vi "process tdms folder.vi"() -> ()   [LabVIEW 2021]
uses:
  NHMFL_Core/Libraries/File/File Format Converter/Format Converter Configuration.ctl
  <vilib>/Utility/TDMS File Viewer/NI_TDMS File Viewer.lvlib
  nanocal_process_tdms_file_control.ctl
panel:
  out "current file index":i32
  out "current file":path
  out "# of files":i32
  out "All Files in Dir":path[](array[path])
  out "ALL channel names":string[](array[string])
  out "new Configuration":T1={"New start time"=nan, "New end time"=nan, "Output file format"=enum."ASCII", "Save ASCII column names"=TRUE, "Prepend binary array size"=FALSE, "buffer size (-1: all)"=100000, "Group"="p", "New dt"=nan, "IGORify column names"=TRUE, "eliminate spaces in col name"=TRUE, "Channels"=[]} {"buffer size (-1: all)" format="%.0p"; "New start time" format="%#_10p"}
  in  "pattern":string="m*_*.tdms"
  in  "Configuration":T1={"New start time"=nan, "New end time"=nan, "Output file format"=enum."ASCII", "Save ASCII column names"=TRUE, "Prepend binary array size"=FALSE, "buffer size (-1: all)"=100000, "Group"="p", "New dt"=nan, "IGORify column names"=TRUE, "eliminate spaces in col name"=TRUE, "Channels"=["jsdhgv", "lsjdfh", "ajlsd"]} {"buffer size (-1: all)" format="%.0p"; "New start time" format="%#_10p"}
  in  "Folder Path":path=path "/Users/arkadyshekhter/Library/CloudStorage/Dropbox/shared_Ali/nanocal-March2020 - RuCl3/March_2020"
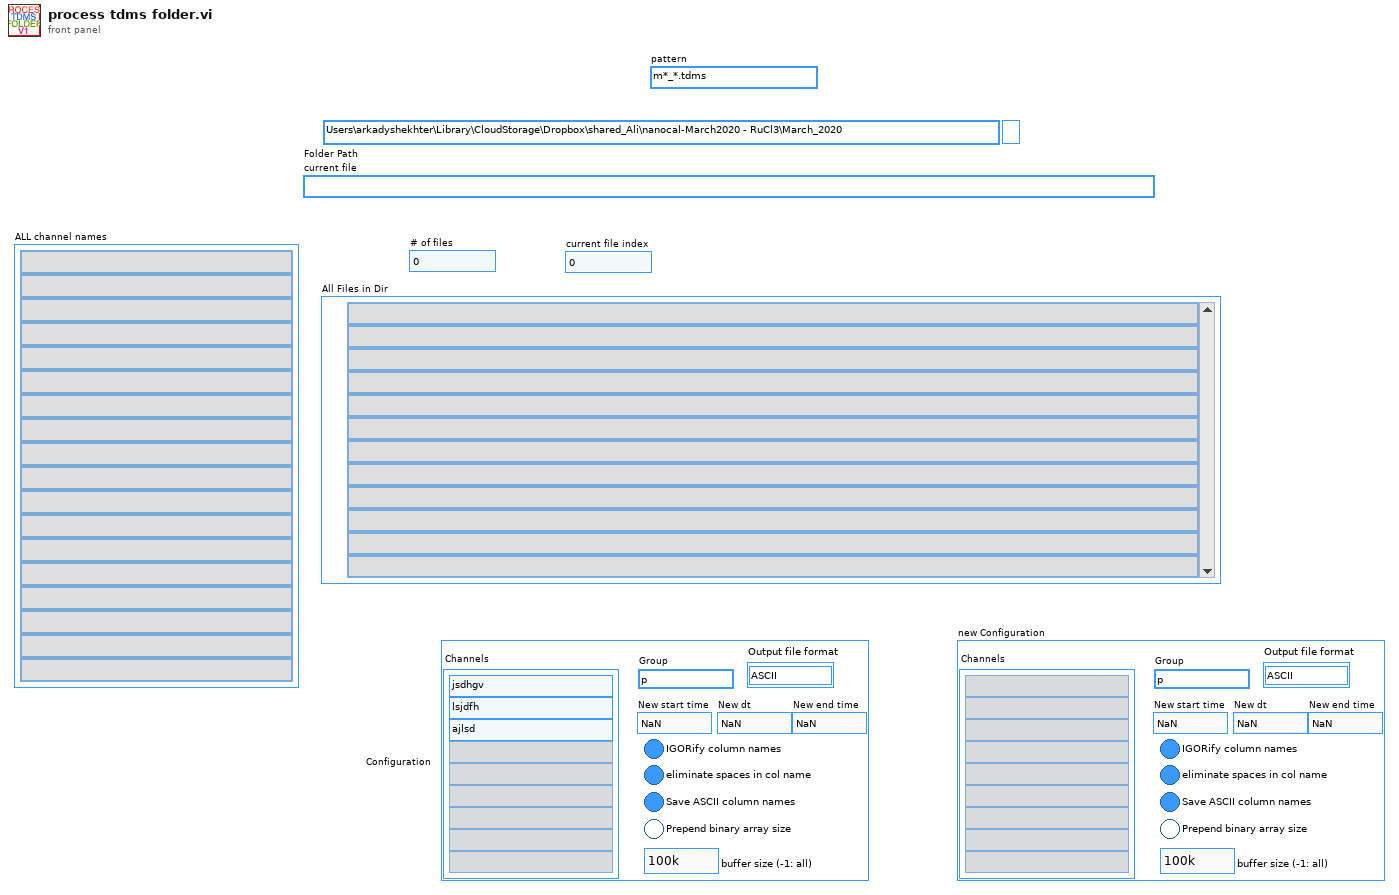
[diagram p1: front panel]
types:
  T1 = typedef "Format Converter Configuration.ctl" = cluster{"New start time":dbl, "New end time":dbl, "Output file format":enum16{"ASCII", "BINARY", "TDMS"}, "Save ASCII column names":bool, "Prepend binary array size":bool, "buffer size (-1: all)":i64, "Group":string, "New dt":dbl, "IGORify column names":bool, "eliminate spaces in col name":bool, "Channels":string[]}
  T2 = typedef "nanocal_process_tdms_file_control.ctl" = enum16{"all fileds", "subset of fields"}
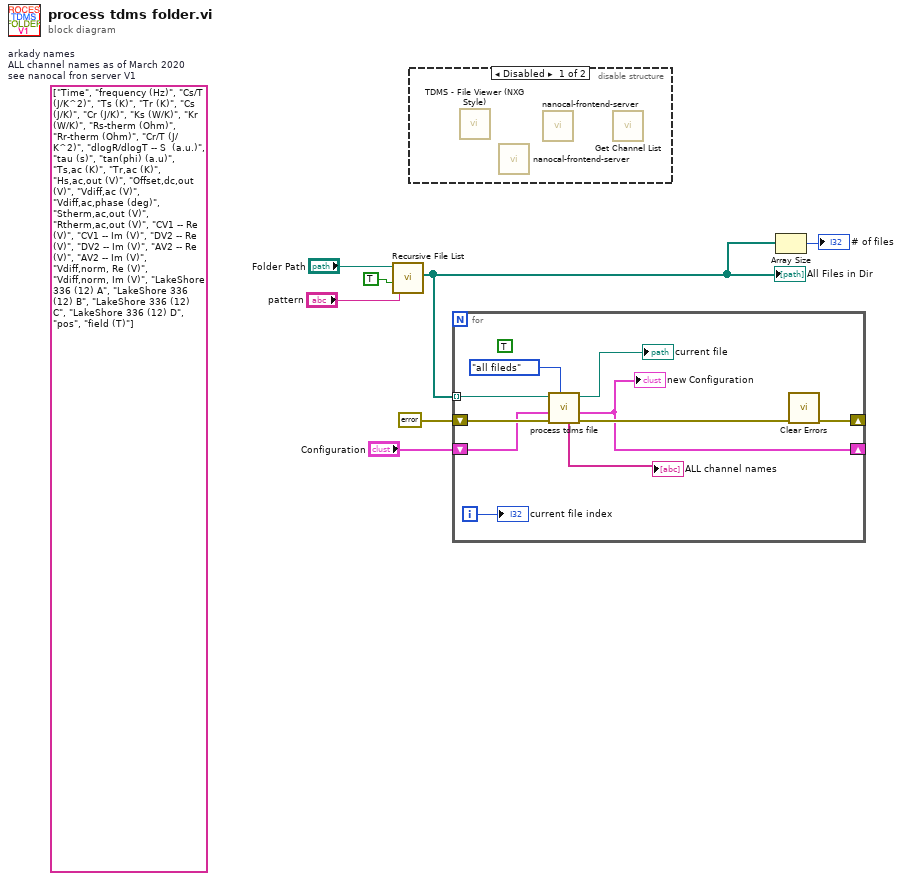
[diagram p0: block diagram]
diagram:
  (unwired) string[] ["Time", "frequency (Hz)", "Cs/T (J/K^2)", "Ts (K)", "Tr (K)", "Cs (J/K)", "Cr (J/K)", "Ks (W/K)", "Kr (W/K)", "Rs-therm (Ohm)", "Rr-therm (Ohm)", "Cr/T (J/K^2)", "dlogR/dlogT -- S  (a.u.)", "tau (s)", "tan(phi) (a.u)", "Ts,ac (K)", "Tr,ac (K)", "Hs,ac,out (V)", "Offset,dc,out (V)", "Vdiff,ac (V)", "Vdiff,ac,phase (deg)", "Stherm,ac,out (V)", "Rtherm,ac,out (V)", "CV1 -- Re (V)", "CV1 -- Im (V)", "DV2 -- Re (V)", "DV2 -- Im (V)", "AV2 -- Re (V)", "AV2 -- Im (V)", "Vdiff,norm, Re (V)", "Vdiff,norm, Im (V)", "LakeShore 336 (12) A", "LakeShore 336 (12) B", "LakeShore 336 (12) C", "LakeShore 336 (12) D", "pos", "field (T)"]  # arkady names ALL channel names as of March 2020 see nanocal fron server V1
  n1 = call <vilib>:"Recursive File List.vi"("pattern"="pattern", "Continue Recursing on Error? (F)"=TRUE, "Folder Path"="Folder Path") -> ("All Files in Dir"=w1:path[])  [unwired: 4 in, 4 out]
  "All Files in Dir" <- w1
  n2 = disable-structure shown="Disabled" {
    frame Disabled {
      n3 = call <vilib>:"TDMS - File Viewer (NXG Style).vi"() -> ()  [unwired: 10 in, 2 out]
      n4 = call "nanocal-frontend-server.vi"() -> ()  [unwired: 12 in]
      n5 = call "nanocal-frontend-server.vi"() -> ()  [unwired: 12 in]
      n6 = call <vilib>:"Get Channel List.vi"() -> ()  [unwired: 5 in, 3 out]
    }
    frame Enabled {
    }
  }
  n7 = for {
    tunnel: w1 -> [w15] mode=indexing
    shift-right: [w17] -> _
    shift-left: errorcluster {"status"=FALSE, "code"=0, "source"=""} ("Error In") -> [w14]
    shift-right: [w10] -> _
    shift-left: "Configuration" -> [w12]
    i -> [w16]
    (unwired) TRUE
    n8 = call "process tdms file.vi"("actions"=nanocal_process_tdms_file_control."all fileds", "Error In"=w14, "Configuration"=w12, "tdms file Path"=w15) -> ("Error Out"=w11:errorcluster, "new Configuration"=w10:T1, "tdms file Path OUT"=→"current file":path, "ALL channel names"=→"ALL channel names":string[])  [unwired: 3 in, 1 out]
    "new Configuration" <- w10
    n9 = call <vilib>:"Clear Errors.vi"("error in (no error)"=w11) -> ("error out"=w17:errorcluster)  [unwired: 5 in, 1 out]
    "current file index" <- w16
  }
  n10 = Array Size(array=w1) -> (size(s)=→"# of files":i32)
